vi "Set_Tunnel_Speed_server.vi"(3 "Tunnel Velocity m/s":dbl min=0.0 max=50.0 format="%.2f", 4 "Rig Name":string, 5 "Mode":T1, 6 "Client Name":string="G3_3 HD") -> (0 "Error String":string, 1 "Settling Time (s)":dbl format="%.2f", 2 "Valid Client":bool)   [LabVIEW 2015]
uses:
  ADAM Client/Sub VIs/ADAM Controls/Tunnel_speed_mode.ctl
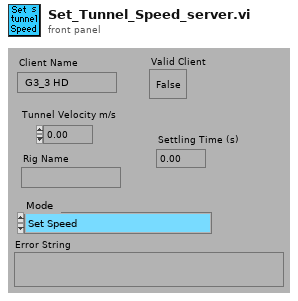
[diagram p1: front panel]
types:
  T1 = typedef "Tunnel_speed_mode.ctl" = enum16{"Set Speed", "Set Speed then wait", "Is tunnel speed allowable?"}
  T2 = typedef "Ch_description_ADAM.ctl" = cluster{"Ch Name":string, "Type":T3, "Function":T4, "Ch State":T5, "Calibration type":T6, "A":dbl, "B":dbl, "C":dbl, "D":dbl, "Comments":string, "Address":T7, "String":string, "Duty":u16}
  T3 = typedef "Module_type_ADAM.ctl" = string
  T4 = typedef "Function_ADAM.ctl" = enum16{"Analogue Input", "Digital Input", "Event counter", "Event rate", "Analogue Output", "Digital Output", "Relay Output"}
  T5 = typedef "Channel_State.ctl" = enum16{"On", "Off", "Always On", "Always Off"}
  T6 = typedef "Calib_type_ADAM.ctl" = enum16{"Raw", "Bx + A", "Cx^2 + Bx + A", "Dx^3 + Cx^2 + Bx + A", "In Band", "Hi-Tec Q", "Hi-Tec M_dot", "Text"}
  T7 = typedef "Address.ctl" = cluster{"Main":i32, "Ch.":i32, "Sub":i32, "Port Name":string}
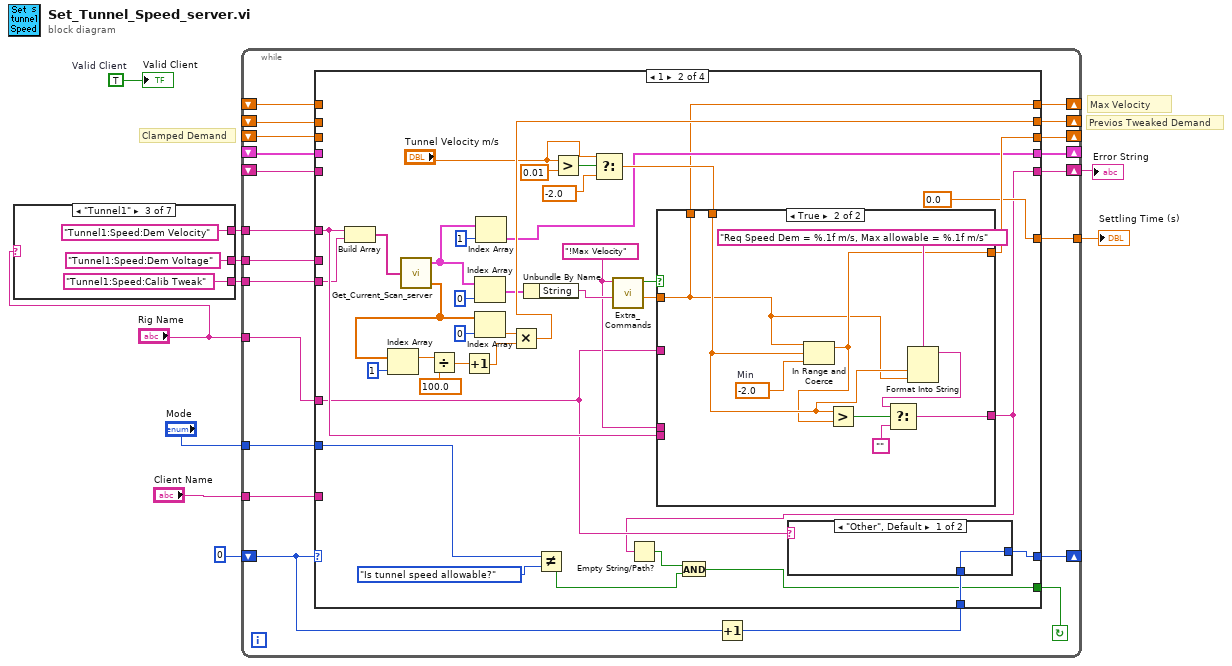
[diagram p0: block diagram]
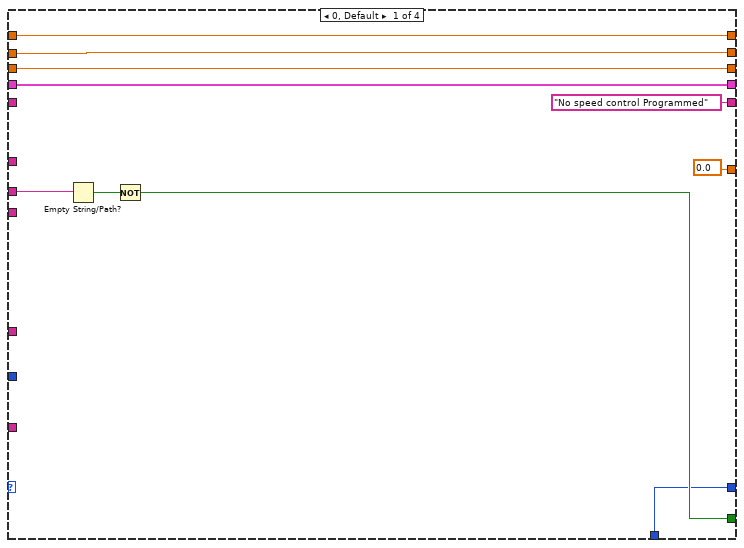
[diagram p2: hidden frame]
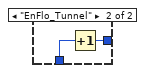
[diagram p3: hidden frame]
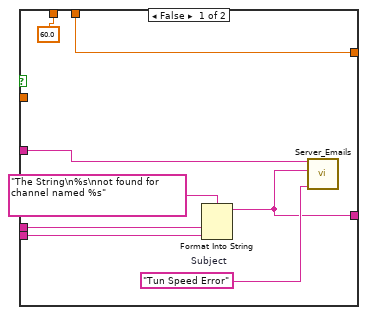
[diagram p4: hidden frame]
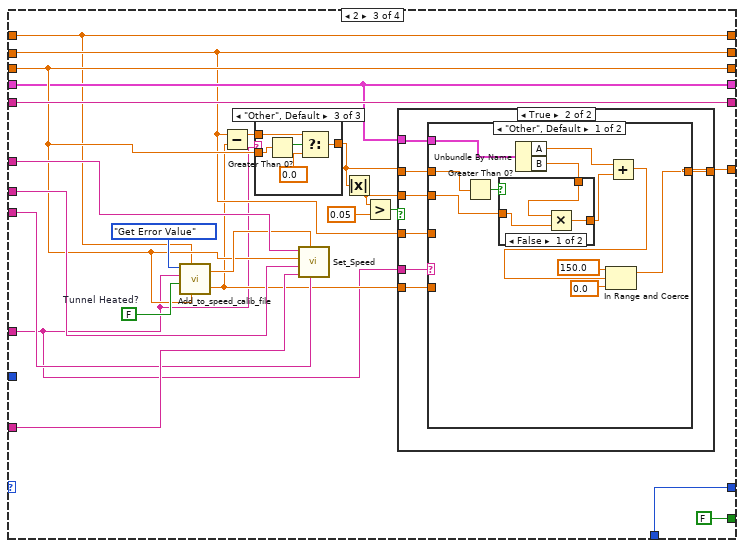
[diagram p5: hidden frame]
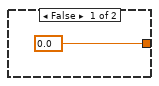
[diagram p8: hidden frame]
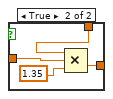
[diagram p9: hidden frame]
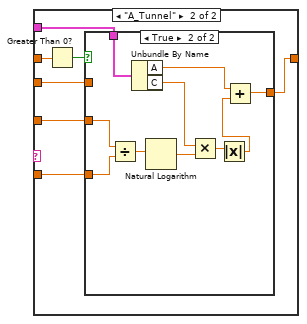
[diagram p10: hidden frame]
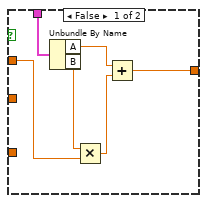
[diagram p11: hidden frame]
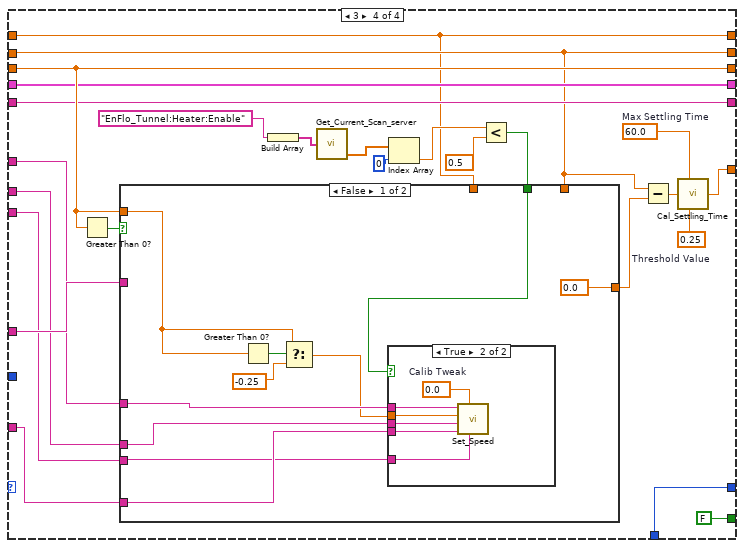
[diagram p12: hidden frame]
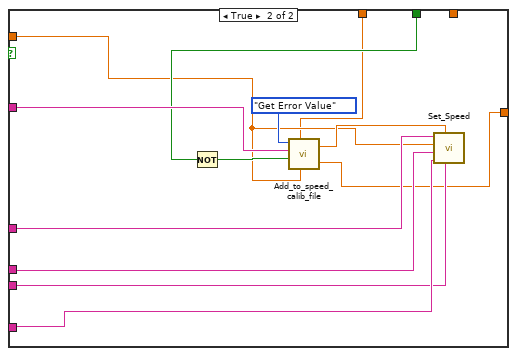
[diagram p14: hidden frame]
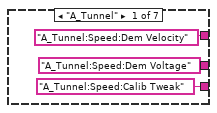
[diagram p15: hidden frame]
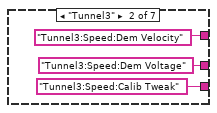
[diagram p16: hidden frame]
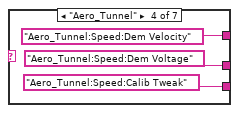
[diagram p17: hidden frame]
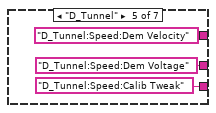
[diagram p18: hidden frame]
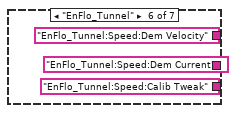
[diagram p19: hidden frame]
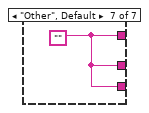
[diagram p20: hidden frame]
diagram:
  w10 = TRUE  # Valid Client
  # "Max Velocity"
  # "Previos Tweaked Demand"
  # "Clamped Demand"
  n1 = case shown="\"Tunnel1\"" "Rig Name" {
    tunnel: ["A_Tunnel:Speed:Dem Velocity" "Tunnel3:Speed:Dem Velocity" "Tunnel1:Speed:Dem Velocity" "Aero_Tunnel:Speed:Dem Velocity" "D_Tunnel:Speed:Dem Velocity" "EnFlo_Tunnel:Speed:Dem Velocity" w29] -> w6
    tunnel: ["A_Tunnel:Speed:Dem Voltage" "Tunnel3:Speed:Dem Voltage" "Tunnel1:Speed:Dem Voltage" "Aero_Tunnel:Speed:Dem Voltage" "D_Tunnel:Speed:Dem Voltage" "EnFlo_Tunnel:Speed:Dem Current" w29] -> w3
    tunnel: ["A_Tunnel:Speed:Calib Tweak" "Tunnel3:Speed:Calib Tweak" "Tunnel1:Speed:Calib Tweak" "Aero_Tunnel:Speed:Calib Tweak" "D_Tunnel:Speed:Calib Tweak" "EnFlo_Tunnel:Speed:Calib Tweak" w29] -> w1
    frame "A_Tunnel" {
    }
    frame "Tunnel3" {
    }
    frame "Tunnel1" {
    }
    frame "Aero_Tunnel" {
    }
    frame "D_Tunnel" {
    }
    frame "EnFlo_Tunnel" {
    }
    frame "Other", Default {
      w29 = ""
    }
  }
  n2 = while {
    shift-left: _ -> [w32]
    shift-right: [w33] -> _
    tunnel: w1 -> [w34]
    shift-left: _ -> [w36]
    shift-right: [w35] -> _
    tunnel: [w37] -> w2
    tunnel: w3 -> [w39]
    shift-left: _ -> [w38]
    shift-right: [w42] -> w5
    shift-left: _ -> [w40]
    shift-right: [w43] -> _
    tunnel: w6 -> [w44]
    shift-left: 0 -> [w47]
    shift-right: [w46] -> _
    tunnel: "Client Name" -> [w49]
    tunnel: "Mode" -> [w50]
    tunnel: "Rig Name" -> [w48]
    shift-right: [w31] -> _
    shift-left: _ -> [w30]
    stop <- w41 continue-if-true
    n3 = Increment(x=w47) -> (x+1=w45:i32)
    n4 = case shown="1" w47 {
      tunnel: w40 -> [w56 _ w129 w210]
      tunnel: w50 -> [_ w89 _ _]
      tunnel: ["No speed control Programmed" w62 w135 w206] -> w42
      tunnel: w49 -> [_ _ w140 w220]
      tunnel: w48 -> [_ w81 w120 w219]
      tunnel: [w57 w84 w138 w211] -> w46
      tunnel: w45 -> [w57 w85 w138 w211]
      tunnel: w44 -> [_ w93 w137 w214]
      tunnel: [w56 w91 w129 w210] -> w43
      tunnel: [w58 w61 FALSE FALSE] -> w41
      tunnel: w39 -> [w60 _ w136 w213]
      tunnel: w38 -> [_ _ w135 w206]
      tunnel: [0.0 ("Settling Time") 0.0 ("Settling Time") w126 w208] -> w37
      tunnel: w36 -> [w54 _ w122 w201]
      tunnel: [w54 w72 w122 w201] -> w35
      tunnel: w34 -> [_ w80 w131 w204]
      tunnel: [w52 w66 w125 w202] -> w33
      tunnel: w32 -> [w52 _ w125 w202]
      tunnel: [w51 w65 w119 w198] -> w31
      tunnel: w30 -> [w51 _ w119 w198]
      frame 0, Default {
        n5 = Empty String/Path?(string/path=w60) -> (empty?=w59:bool)
        n6 = Not(x=w59) -> (.not. x?=w58:bool)
      }
      frame 1 {
        w94 = "!Max Velocity" ("Command")
        n7 = Build Array(w93, w80) -> (w98:string[])
        n8 = call "Get_Current_Scan_server.vi"("Desired Channels"=w98) -> ("Ch Description Array"=w67:T2[], "Numerical Values"=w78:dbl[])  [unwired: 1 out]
        n9 = Index Array(array=w78, index=1 ("Index")) -> (element=w77:dbl)
        n10 = Divide(x=w77, y=100.0) -> (x/y=w75:dbl)
        n11 = Increment(x=w75) -> (x+1=w73:dbl)
        n12 = Index Array(array=w67, index=0 ("Index")) -> (element=w69:T2)
        n13 = Index Array(array=w78, index=0 ("Index")) -> (element=w74:dbl)
        n14 = Index Array(array=w67, index=1 ("Index")) -> (element=w66:T2)
        n15 = Multiply(x=w74, y=w73) -> (x*y=w72:dbl)
        n16 = Unbundle By Name(w69) -> ("String"=w96:string)
        n17 = Not Equal?(x=w89, y=Tunnel_speed_mode."Is tunnel speed allowable?" ("Mode")) -> (x != y?=w63:bool)
        n18 = Greater?(x="Tunnel Velocity m/s", y=0.01) -> (0:w88:bool)
        n19 = Select(t="Tunnel Velocity m/s", s=w88, f=-2.0 ("t")) -> (s? t:f=w86:dbl)
        n20 = call "Extra_Commands.vi"("String to Search"=w96, "Command"=w94) -> ("Numeric Value"=w92:dbl, "Command Found"=w95:bool)  [unwired: 1 in, 3 out]
        n21 = case shown="True" w95 {
          tunnel: w81 -> [w103 _]
          tunnel: w94 -> [w108 _]
          tunnel: w93 -> [w107 _]
          tunnel: w92 -> [_ w110]
          tunnel: w86 -> [w105 w112]
          tunnel: [w105 w111] -> w91
          tunnel: [w104 w114] -> w62
          tunnel: [60.0 ("Numeric Value") w110] -> w65
          frame False {
            w109 = "Tun Speed Error"  # Subject
            n22 = Format Into String(format string="The String\n%s\nnot found for channel named %s" ("Format String"), w108, w107) -> (resulting string=w104:string)  [unwired: 2 in, 1 out]
            n23 = call "Server_Emails.vi"("Client Name Contains"=w103, "Message"=w104, "Subject"=w109) -> ()  [unwired: 2 in, 3 out]
          }
          frame True {
            w118 = -2.0  # Min
            n24 = In Range and Coerce(upper limit=w110, x=w112, lower limit=w118) -> (coerced(x)=w111:dbl)  [unwired: 1 out]
            n25 = Greater?(x=w112, y=w111) -> (0:w113:bool)
            n26 = Format Into String(format string="Req Speed Dem = %.1f m/s, Max allowable = %.1f m/s", w112, w110) -> (resulting string=w116:string)  [unwired: 2 in, 1 out]
            n27 = Select(t=w116, s=w113, f="") -> (s? t:f=w114:string)
          }
        }
        n28 = Empty String/Path?(string/path=w62) -> (empty?=w64:bool)
        n29 = And(x=w64, y=w63) -> (x .and. y?=w61:bool)
        n30 = case shown="\"Other\", Default" w81 {
          tunnel: w85 -> [w99 w101]
          tunnel: [w99 w100] -> w84
          frame "Other", Default {
          }
          frame "EnFlo_Tunnel" {
            n31 = Increment(x=w101) -> (x+1=w100:i32)
          }
        }
      }
      frame 2 {
        w132 = FALSE  # Tunnel Heated?
        n32 = call "Add_to_speed_calib_file.vi"("Desired Velocity"=w129, "Max Velocity"=w119, "Tunnel Heated?"=w132, "Rig Name"=w120, "Mode"=enum16{"Add Row", "Get Error Value"}."Get Error Value") -> ("Tweaked Demand"=w121:dbl, "Calib Tweak %"=w130:dbl)  [unwired: 1 in]
        n33 = Subtract(x=w122, y=w121) -> (x-y=w133:dbl)
        n34 = case shown="\"Other\", Default" w120 {
          tunnel: w133 -> [w141 w142 w147]
          tunnel: w129 -> [_ _ w145]
          tunnel: [w141 w142 w144] -> w124
          frame "Tunnel1" {
          }
          frame "Tunnel3" {
          }
          frame "Other", Default {
            n35 = Greater Than 0?(x=w145) -> (x > 0?=w143:bool)
            n36 = Select(t=w147, s=w143, f=0.0) -> (s? t:f=w144:dbl)
          }
        }
        n37 = call "Set_Speed.vi"("Channel Name (Calib Tweak)"=w131, "Calib Tweak"=w130, "Client Name"=w140, "Channel Name (Volts/Amps)"=w136, "Demanded Velocity"=w129, "Channel Name (Velocity)"=w137) -> ()  [unwired: 1 in, 4 out]
        n38 = Absolute Value(x=w124) -> (abs(x)=w123:dbl)
        n39 = Greater?(x=w123, y=0.05) -> (0:w127:bool)
        n40 = case shown="True" w127 {
          tunnel: w125 -> [_ w155]
          tunnel: [0.0 w152] -> w126
          tunnel: w124 -> [_ w154]
          tunnel: w123 -> [_ w153]
          tunnel: w120 -> [_ w151]
          tunnel: w122 -> [_ w150]
          tunnel: w121 -> [_ w149]
          frame False {
          }
          frame True {
            n41 = case shown="\"Other\", Default" w151 {
              tunnel: w155 -> [w166 w177]
              tunnel: w154 -> [w161 w179]
              tunnel: w153 -> [w157 w178]
              tunnel: [w156 w176] -> w152
              tunnel: w150 -> [_ w175]
              tunnel: w149 -> [_ w174]
              frame "Other", Default {
                n42 = Greater Than 0?(x=w161) -> (x > 0?=w160:bool)
                n43 = Unbundle By Name(w166) -> ("A"=w165:dbl, "B"=w159:dbl)
                n44 = case shown="False" w160 {
                  tunnel: [w169 w170] -> w158
                  tunnel: w159 -> [w168 w173]
                  tunnel: w157 -> [w167 w172]
                  frame False {
                    n45 = Multiply(x=w168, y=w167) -> (x*y=w169:dbl)
                  }
                  frame True {
                    n46 = Compound Arithmetic op=MULTIPLY(w173, w172, 1.35 ("Min")) -> (w170:dbl)
                  }
                }
                n47 = Add(x=w165, y=w158) -> (x+y=w162:dbl)
                n48 = In Range and Coerce(upper limit=150.0 ("Max"), x=w162, lower limit=0.0 ("Min")) -> (coerced(x)=w156:dbl)  [unwired: 1 out]
              }
              frame "A_Tunnel" {
                n49 = Greater Than 0?(x=w179) -> (x > 0?=w180:bool)
                n50 = case shown="True" w180 {
                  tunnel: w178 -> [w182 _]
                  tunnel: w177 -> [w186 w196]
                  tunnel: [w181 w187] -> w176
                  tunnel: w175 -> [_ w194]
                  tunnel: w174 -> [_ w193]
                  frame False {
                    n51 = Unbundle By Name(w186) -> ("A"=w185:dbl, "B"=w183:dbl)
                    n52 = Multiply(x=w183, y=w182) -> (x*y=w184:dbl)
                    n53 = Add(x=w185, y=w184) -> (x+y=w181:dbl)
                  }
                  frame True {
                    n54 = Divide(x=w194, y=w193) -> (x/y=w195:dbl)
                    n55 = Unbundle By Name(w196) -> ("A"=w188:dbl, "C"=w191:dbl)
                    n56 = Natural Logarithm(1:w195) -> (0:w192:dbl)
                    n57 = Multiply(x=w191, y=w192) -> (x*y=w190:dbl)
                    n58 = Absolute Value(x=w190) -> (abs(x)=w189:dbl)
                    n59 = Add(x=w188, y=w189) -> (x+y=w187:dbl)
                  }
                }
              }
            }
          }
        }
      }
      frame 3 {
        w209 = 0.25  # Threshold Value
        w197 = 60.0  # Max Settling Time
        n60 = Greater Than 0?(x=w210) -> (x > 0?=w221:bool)
        n61 = Build Array("EnFlo_Tunnel:Heater:Enable") -> (w200:string[])
        n62 = call "Get_Current_Scan_server.vi"("Desired Channels"=w200) -> ("Numerical Values"=w199:dbl[])  [unwired: 2 out]
        n63 = Index Array(array=w199, index=0) -> (element=w215:dbl)
        n64 = Less?(x=w215, y=0.5) -> (x < y?=w205:bool)
        n65 = case shown="False" w221 {
          tunnel: w210 -> [w229 w239]
          tunnel: w214 -> [w228 w249]
          tunnel: w213 -> [w226 w248]
          tunnel: w220 -> [w225 w247]
          tunnel: w219 -> [_ w246]
          tunnel: w205 -> [w224 w244]
          tunnel: [0.0 w240] -> w203
          tunnel: w204 -> [w222 w242]
          tunnel: w201 -> [_ _]
          tunnel: w198 -> [_ w238]
          frame False {
            n66 = Greater Than 0?(x=w229) -> (x > 0?=w231:bool)
            n67 = Select(t=w229, s=w231, f=-0.25 ("t")) -> (s? t:f=w227:dbl)
            n68 = case shown="True" w224 {
              tunnel: w228 -> [_ w237]
              tunnel: w227 -> [_ w236]
              tunnel: w226 -> [_ w235]
              tunnel: w225 -> [_ w234]
              tunnel: w222 -> [_ w233]
              frame False {
              }
              frame True {
                w232 = 0.0  # Calib Tweak
                n69 = call "Set_Speed.vi"("Channel Name (Calib Tweak)"=w233, "Calib Tweak"=w232, "Client Name"=w234, "Channel Name (Volts/Amps)"=w235, "Demanded Velocity"=w236, "Channel Name (Velocity)"=w237) -> ()  [unwired: 1 in, 4 out]
              }
            }
          }
          frame True {
            n70 = Not(x=w244) -> (.not. x?=w243:bool)
            n71 = call "Add_to_speed_calib_file.vi"("Desired Velocity"=w239, "Max Velocity"=w238, "Tunnel Heated?"=w243, "Rig Name"=w246, "Mode"=enum16{"Add Row", "Get Error Value"}."Get Error Value") -> ("Tweaked Demand"=w240:dbl, "Calib Tweak %"=w241:dbl)  [unwired: 1 in]
            n72 = call "Set_Speed.vi"("Channel Name (Calib Tweak)"=w242, "Calib Tweak"=w241, "Client Name"=w247, "Channel Name (Volts/Amps)"=w248, "Demanded Velocity"=w239, "Channel Name (Velocity)"=w249) -> ()  [unwired: 1 in, 4 out]
          }
        }
        n73 = Subtract(x=w201, y=w203) -> (x-y=w207:dbl)
        n74 = call "Cal_Settling_Time.vi"("Max Settling Time"=w197, "Speed Tweak (m/s)"=w207, "Threshold Value"=w209) -> ("Required Settling Time"=w208:dbl)  [unwired: 2 out]
      }
    }
  }
  "Error String" <- w5
  "Settling Time (s)" <- w2
  "Valid Client" <- w10
